vi "Configure Alarms.vi"(6 "Boolean Alarm Controls":T2, 8 "error in (no error)":errorcluster, 9 "Alarm Limits":T1 {"Deadband (0.0000)" min=0.0 max=9999.9 step=0.0001 format="%.4f"; "Low Value (0.0000)" min=-9999.9 max=9999.9 step=0.0001 format="%.4f"; "High Value (0.0000)" min=-9999.9 max=9999.9 step=0.0001 format="%.4f"}, 10 "Input (0)":i32 min=0 max=7 step=1, 11 "LS218 in":refnum<class "LS218.lvclass">) -> (0 "error out":errorcluster, 3 "LS218 out":refnum<class "LS218.lvclass">)   [LabVIEW 2015, in "LS218.lvlib" / "LS218.lvclass"]
doc: "This VI configures all alarm functions for the selected input. Alarm functions include source, on/off, high value, low value, deadband, and latching parameters. This VI also enables/disables the system beeper, this control applies to all inputs."
uses:
  LS218.lvclass
  LS218.lvclass/LS218.ctl
  <instrlib>/Lake Shore Cryotronics 218/Lake Shore Cryotronics 218.lvlib
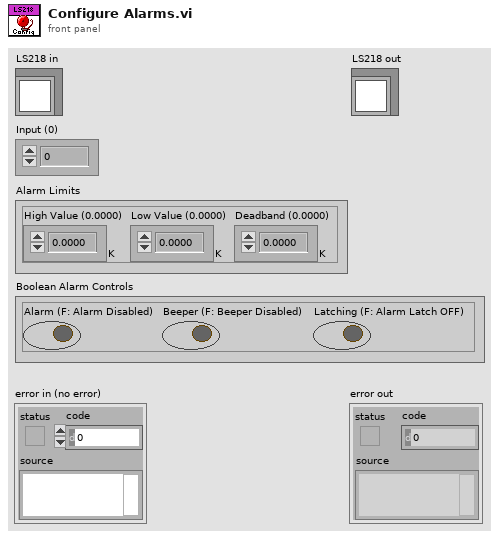
[diagram p1: front panel]
types:
  T1 = cluster{"High Value (0.0000)":dbl[unit], "Low Value (0.0000)":dbl[unit], "Deadband (0.0000)":dbl[unit]}
  T2 = cluster{"Alarm (F: Alarm Disabled)":bool, "Beeper (F: Beeper Disabled)":bool, "Latching (F: Alarm Latch OFF)":bool}
  T3 = cluster{"High Value (0.0000)":dbl, "Low Value (0.0000)":dbl, "Deadband (0.0000)":dbl}
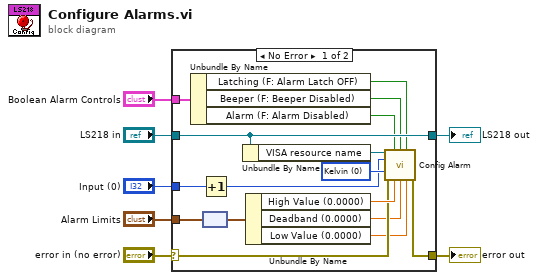
[diagram p0: block diagram]
diagram:
  n1 = case shown="No Error" "error in (no error)" {
    selector: "error in (no error)" -> [w13 w25]
    tunnel: [w12 w25] -> w6
    tunnel: [w22 w24] -> w4
    tunnel: "LS218 in" -> [w22 w24]
    tunnel: "Input (0)" -> [w20 _]
    tunnel: "Boolean Alarm Controls" -> [w19 _]
    tunnel: "Alarm Limits" -> [w15 _]
    frame No Error {
      w23 = u16 0 items=["Kelvin", "Celsius", "Sensor Units", "Linear Data"] ("Alarm Source (0:Kelvin)")
      n2 = Unbundle By Name(w19) -> ("Latching (F: Alarm Latch OFF)"=w16:bool, "Beeper (F: Beeper Disabled)"=w17:bool, "Alarm (F: Alarm Disabled)"=w18:bool)
      n3 = Increment(x=w20) -> (x+1=w10:i32)
      n4 = node(w15) -> (w11:T3)
      n5 = Unbundle By Name(w22) -> ("VISA resource name"=w21:refnum<visa-resource-name>)
      n6 = Unbundle By Name(w11) -> ("High Value (0.0000)"=w14:dbl, "Deadband (0.0000)"=w9:dbl, "Low Value (0.0000)"=w8:dbl)
      n7 = call <instrlib>:"Config Alarm.vi"("VISA resource name"=w21, "Alarm (F: Alarm Disabled)"=w18, "Beeper (F: Beeper Disabled)"=w17, "Latching (F: Alarm Latch OFF)"=w16, "Input (1)"=w10, "Alarm Source (0:Kelvin)"=w23, "error in (no error)"=w13, "High Value (0.0000)"=w14, "Deadband (0.0000)"=w9, "Low Value (0.0000)"=w8) -> ("error out"=w12:errorcluster)  [unwired: 4 in, 1 out]
    }
    frame Error {
    }
  }
  "error out" <- w6
  "LS218 out" <- w4
